vi "SW_STATUS.vi"(7 "IP":string="192.168.23.100", 8 "error in":errorcluster, 10 "PORT":dbl=1.0 min=1.0 max=4.0 step=1.0, 11 "MASTER":dbl=1.0 min=1.0 max=10.0 step=1.0) -> (0 "error out 2":errorcluster, 1 "ON":bool[](array[boolean]), 2 "PWM (%)":dbl, 3 "ON":i32, 5 "Chart":i32(graph))   [LabVIEW 2022 SP3]
uses:
  <vilib>/JDP Science/JSONtext/Next JSON Value.vi
  <vilib>/JDP Science/JSONtext/String Subset.vi
  <vilib>/JDP Science/JSONtext/Parsing/Advance past next JSON Value (inlined COPY).vi
  <vilib>/JDP Science/JSONtext/Parsing/Advance past whitespace.vi
  <vilib>/JDP Science/JSONtext/Parsing/Advance past String.vi
  <vilib>/JDP Science/JSONtext/Parsing/Advance past Number.vi
  <vilib>/JDP Science/JSONtext/Parsing/Advance past Line Ending.vi
  <vilib>/JDP Science/JSONtext/Parsing/Parse Full Path or Item Name.vi
  <vilib>/JDP Science/JSONtext/Parsing/Advance past Array.vi
  <vilib>/JDP Science/JSONtext/Parsing/Advance past Object.vi
  <vilib>/JDP Science/JSONtext/support/Error Cluster From Code.vi
  <vilib>/JDP Science/JSONtext/Offset/Find Item Locations by Path.vi
  <vilib>/JDP Science/JSONtext/JSONtext.lvlib
  <vilib>/NI/Advanced HTTP Client/Session.lvclass
panel:
  out "body":string
  # "Smart conn status on /off"
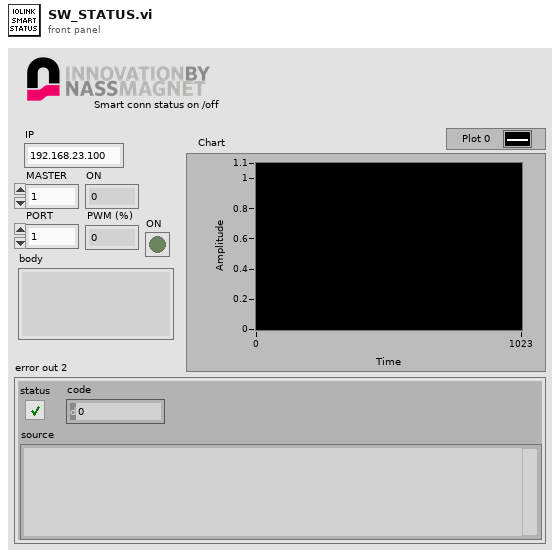
[diagram p1: front panel]
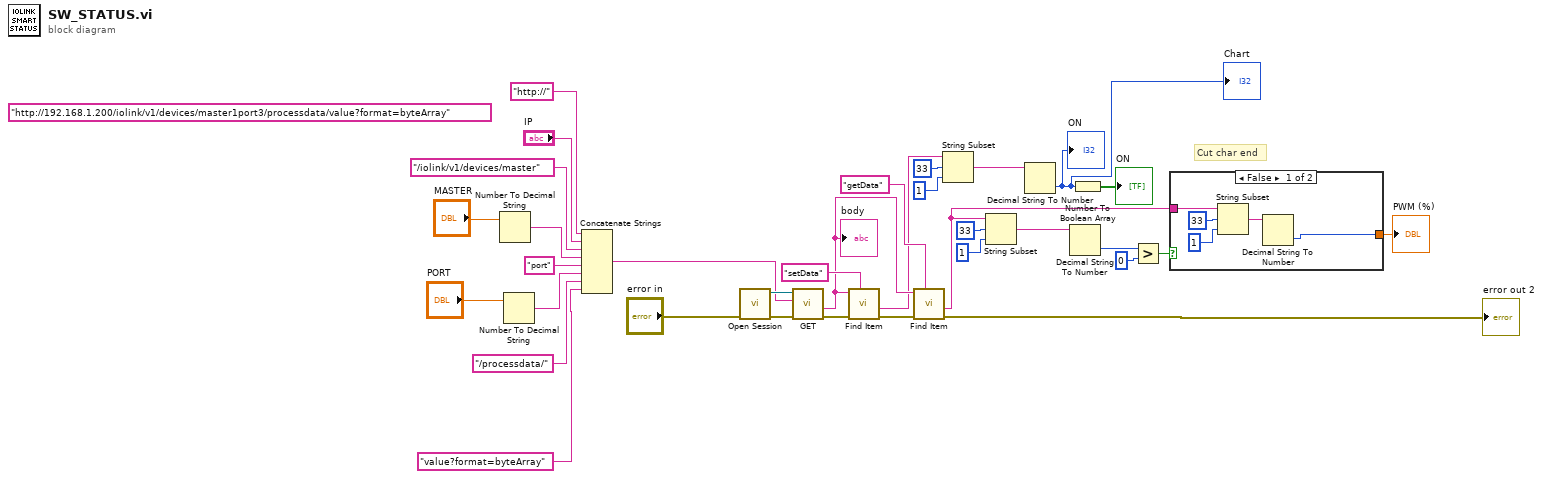
[diagram p0: block diagram]
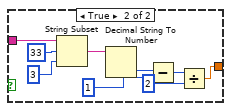
[diagram p2: hidden frame]
diagram:
  (unwired) "http://192.168.1.200/iolink/v1/devices/master1port3/processdata/value?format=byteArray" ("url")
  # "Cut char end"
  n1 = Number To Decimal String(number="MASTER") -> (decimal integer string=w25:string)  [unwired: 1 in]
  n2 = Number To Decimal String(number="PORT") -> (decimal integer string=w22:string)  [unwired: 1 in]
  n3 = Concatenate Strings("http://" ("string"), "IP", "/iolink/v1/devices/master" ("string"), w25, "port" ("string"), w22, "/processdata/" ("string"), "value?format=byteArray" ("string")) -> (w26:string)
  n4 = call <vilib>:"Open Session.vi"("error in"="error in") -> ("error out"=w33:errorcluster, "session"=w34:refnum<class "Session.lvclass">)  [unwired: 9 in]
  n5 = call <vilib>:"GET.vi"("error in"=w33, "url"=w26, "session in"=w34) -> ("error out"=w4:errorcluster, "body"=w18:string)  [unwired: 4 in, 3 out]
  "body" <- w18
  n6 = call <vilib>:"Find Item.vi"("$Path or Item Name"="setData", "error in (no error)"=w4, "JSON"=w18) -> ("error out"=w3:errorcluster, "<JSON>"=w17:string)  [unwired: 5 in, 2 out]
  n7 = call <vilib>:"Find Item.vi"("$Path or Item Name"="getData", "error in (no error)"=w3, "JSON"=w18) -> ("error out"=→"error out 2":errorcluster, "<JSON>"=w11:string)  [unwired: 5 in, 2 out]
  n8 = String Subset(string=w17, offset (0)=33, length (rest)=1 ("length (rest)")) -> (substring=w7:string)
  n9 = String Subset(string=w11, offset (0)=33, length (rest)=1 ("length (rest)")) -> (substring=w9:string)
  n10 = Decimal String To Number(string=w7) -> (number=w5:i32)  [unwired: 2 in, 1 out]
  "ON" <- w5
  "Chart" <- w5
  n11 = Decimal String To Number(string=w9) -> (number=w8:i32)  [unwired: 2 in, 1 out]
  n12 = Number To Boolean Array(number=w5) -> (Boolean array=→"ON":bool[])
  n13 = Greater?(x=w8, y=0) -> (0:w12:bool)
  n14 = case shown="False" w12 {
    tunnel: w11 -> [w37 w46]
    tunnel: [w35 w40] -> w1
    frame False {
      n15 = String Subset(string=w37, offset (0)=33, length (rest)=1 ("length (rest)")) -> (substring=w36:string)
      n16 = Decimal String To Number(string=w36) -> (number=w35:i32)  [unwired: 2 in, 1 out]
    }
    frame True {
      n17 = String Subset(string=w46, offset (0)=33, length (rest)=3 ("length (rest)")) -> (substring=w45:string)
      n18 = Decimal String To Number(string=w45) -> (number=w44:i32)  [unwired: 2 in, 1 out]
      n19 = Subtract(x=w44, y=1) -> (x-y=w42:i32)
      n20 = Divide(x=w42, y=2) -> (x/y=w40:dbl)
    }
  }
  "PWM (%)" <- w1
